vi "OnOff — копия.vi"(0 "setpoint":dbl step=0.01 format="%.2f", 1 "X1(SetState)":i32, 2 "reinitialize? (F)":bool, 5 "process variable":dbl step=0.01 format="%.2f", 7 "PID gains":T2={"proportional gain (Kc)"=1.0, "integral time (Ti, s)"=10.0, "derivative time (Td, s)"=1.0} {"derivative time (Td, s)" format="%.3f"; "integral time (Ti, s)" format="%.3f"; "proportional gain (Kc)" format="%.3f"}, 9 "manual control":dbl format="%.2f", 12 "output param":T1={"output high"=100.0, "alr value"=0.0, "output low"=0.0, "output rate (EGU/s)"=1.0, "dt (s)"=-1.0} {"dt (s)" format="%.3f"; "output rate (EGU/s)" format="%.2f"; "alr value" format="%.2f"; "output low" format="%.2f"; "output high" format="%.2f"}) -> (4 "output":dbl format="%.2f", 10 "dt out (s)":dbl format="%.3f")   [LabVIEW 2015]
uses:
  Userlib.lvlib
panel:
  # "Входы\nX1(SetState) заданное состояние\n     0 – аварийное значение\n     1 – минимум\n     2 – стоп\n     3 – ручной\n     4 – автомат\n     5 – максимум"
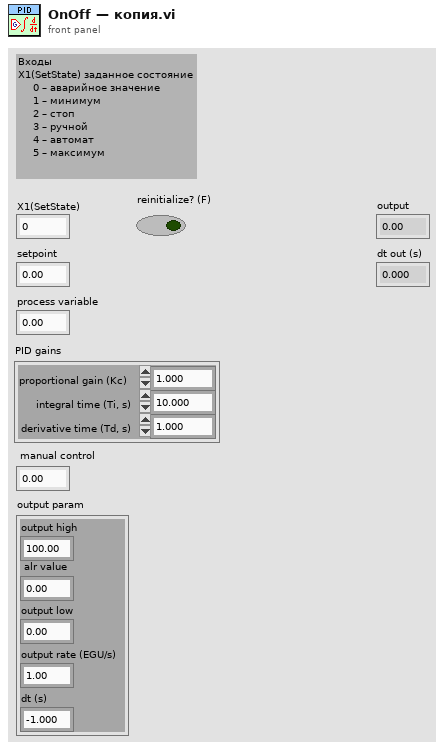
[diagram p1: front panel]
types:
  T1 = cluster{"output high":dbl, "alr value":dbl, "output low":dbl, "output rate (EGU/s)":dbl, "dt (s)":dbl}
  T2 = cluster{"proportional gain (Kc)":dbl, "integral time (Ti, s)":dbl, "derivative time (Td, s)":dbl}
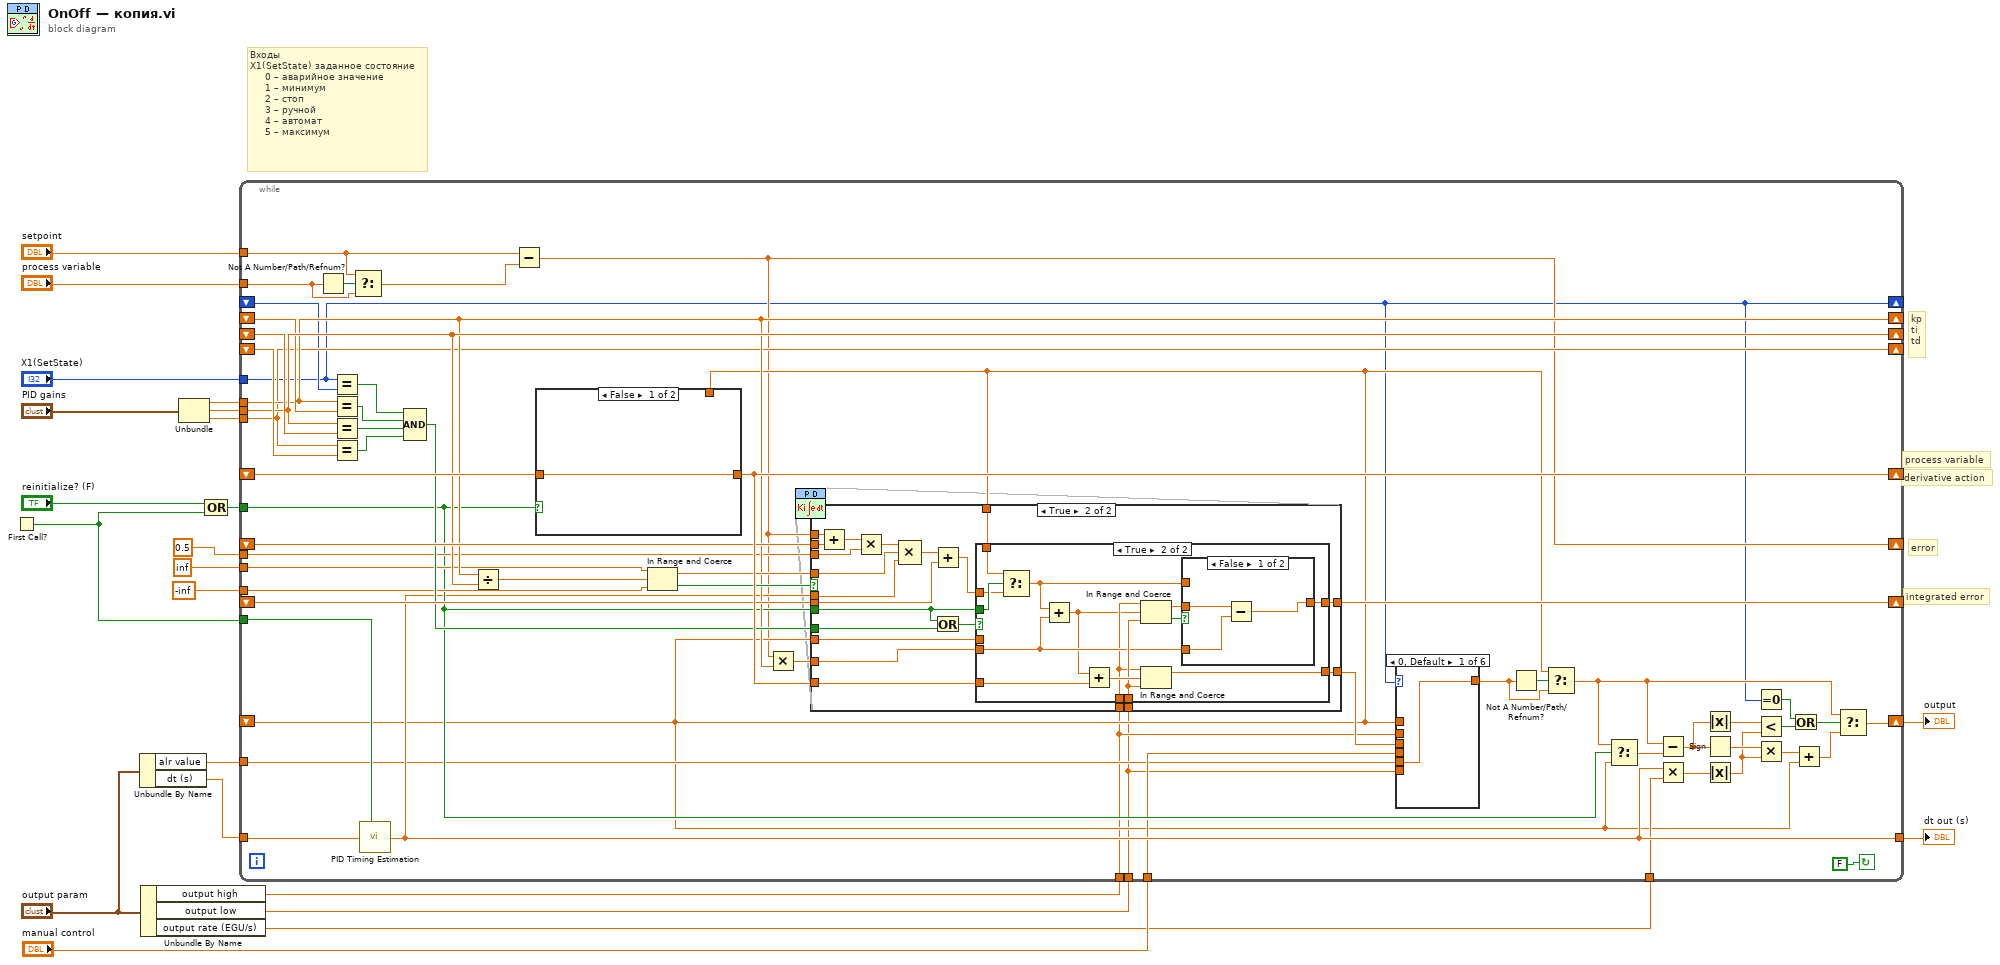
[diagram p0: block diagram]
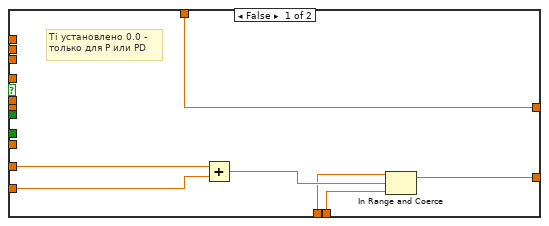
[diagram p2: hidden frame]
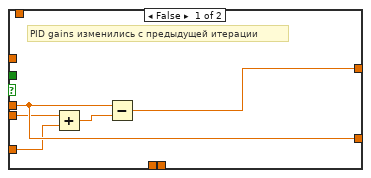
[diagram p3: hidden frame]
diagram:
  # "derivative action"
  # "process variable"
  # "kp\nti\ntd"
  # "error"
  # "integrated error"
  # "Входы\nX1(SetState) заданное состояние\n     0 – аварийное значение\n     1 – минимум\n     2 – стоп\n     3 – ручной\n     4 – автомат\n     5 – максимум"
  n1 = First Call?() -> (First Call?: T/F=w22:bool)
  n2 = Unbundle By Name("output param") -> ("alr value"=w6:dbl, "dt (s)"=w5:dbl)
  n3 = Unbundle By Name("output param") -> ("output high"=w14:dbl, "output low"=w15:dbl, "output rate (EGU/s)"=w1:dbl)
  n4 = Unbundle("PID gains") -> ("proportional gain (Kc)"=w11:dbl, "integral time (Ti, s)"=w12:dbl, "derivative time (Td, s)"=w13:dbl)
  n5 = Compound Arithmetic op=OR("reinitialize? (F)", w22) -> (w10:bool)
  n6 = while {
    tunnel: w10 -> [w49]
    shift-right: [w62] -> _
    shift-left: _ -> [w63]
    shift-right: [w64] -> _
    shift-left: _ -> [w78]
    shift-right: [w57] -> _
    shift-left: _ -> [w79]
    tunnel: w11 -> [w62]
    tunnel: w12 -> [w64]
    tunnel: w13 -> [w57]
    tunnel: w5 -> [w55]
    tunnel: w14 -> [w28]
    tunnel: w15 -> [w27]
    tunnel: "process variable" -> [w23]
    shift-right: [w74] -> _
    shift-left: _ -> [w68]
    shift-right: [w31] -> _
    shift-left: _ -> [w73]
    shift-right: [w72] -> _
    shift-left: _ -> [w71]
    tunnel: 0.5 ("y") -> [w61]
    tunnel: inf ("upper limit") -> [w59]
    tunnel: -inf ("lower limit") -> [w60]
    tunnel: w22 -> [w56]
    tunnel: [w48] -> w9
    tunnel: "manual control" -> [w38]
    tunnel: w1 -> [w47]
    shift-right: [w41] -> w7
    shift-left: _ -> [w34]
    tunnel: w6 -> [w36]
    tunnel: "X1(SetState)" -> [w29]
    shift-right: [w29] -> _
    shift-left: _ -> [w35]
    tunnel: "setpoint" -> [w24]
    stop <- FALSE continue-if-true
    n7 = Not A Number/Path/Refnum?(number/path/refnum=w23) -> (NaN/Path/Refnum?=w25:bool)
    n8 = Equal?(x=w29, y=w35) -> (x = y?=w30:bool)
    n9 = Equal?(x=w62, y=w63) -> (x = y?=w76:bool)
    n10 = Equal?(x=w64, y=w78) -> (x = y?=w75:bool)
    n11 = Equal?(x=w57, y=w79) -> (x = y?=w77:bool)
    n12 = Select(t=w24, s=w25, f=w23) -> (s? t:f=w26:dbl)
    n13 = call "PID Timing Estimation.vi"("R"=w56, "dt (s) in"=w55) -> ("dt (s) out"=w48:dbl)  [unwired: 7 in]
    n14 = Compound Arithmetic op=AND(w30, w76, w75, w77) -> (w65:bool)
    n15 = Divide(x=w62, y=w64) -> (x/y=w67:dbl)
    n16 = Subtract(x=w24, y=w26) -> (x-y=w31:dbl)
    n17 = case shown="False" w49 {
      tunnel: [w131 w132] -> w74
      tunnel: w68 -> [w131 _]
      tunnel: w34 -> [_ w132]
      frame False {
      }
      frame True {
      }
    }
    n18 = In Range and Coerce(upper limit=w59, x=w67, lower limit=w60) -> (coerced(x)=w70:dbl, In Range?=w69:bool)
    n19 = Multiply(x=w31, y=w62) -> (x*y=w66:dbl)
    n20 = case shown="True" w69 {
      tunnel: w31 -> [_ w106]
      tunnel: w73 -> [_ w107]
      tunnel: w71 -> [_ w102]
      tunnel: [w80 w97] -> w72
      tunnel: w70 -> [_ w95]
      tunnel: w66 -> [w85 w100]
      tunnel: [w86 w96] -> w39
      tunnel: w34 -> [_ w98]
      tunnel: w74 -> [w84 w94]
      tunnel: w49 -> [_ w93]
      tunnel: w65 -> [_ w92]
      tunnel: w48 -> [_ w91]
      tunnel: w28 -> [w82 w89]
      tunnel: w27 -> [w81 w90]
      tunnel: w61 -> [_ w88]
      tunnel: w34 -> [w80 w87]
      frame False {
        # "Ti установлено 0.0 -\nтолько для P или PD"
        n21 = Add(x=w85, y=w84) -> (x+y=w83:dbl)
        n22 = In Range and Coerce(upper limit=w82, x=w83, lower limit=w81) -> (coerced(x)=w86:dbl)  [unwired: 1 out]
      }
      frame True {
        n23 = Add(x=w106, y=w107) -> (x+y=w105:dbl)
        n24 = Multiply(x=w105, y=w88) -> (x*y=w104:dbl)
        n25 = Compound Arithmetic op=MULTIPLY(w104, w95, w91) -> (w103:dbl)
        n26 = Add(x=w103, y=w102) -> (x+y=w101:dbl)
        n27 = Or(x=w93, y=w92) -> (x .or. y?=w99:bool)
        n28 = case shown="True" w99 {
          tunnel: w101 -> [_ w113]
          tunnel: w100 -> [w110 w119]
          tunnel: w98 -> [w112 _]
          tunnel: w93 -> [_ w116]
          tunnel: [w111 w121] -> w97
          tunnel: [w112 w125] -> w96
          tunnel: w94 -> [w109 w124]
          tunnel: w90 -> [_ w123]
          tunnel: w89 -> [_ w118]
          tunnel: w87 -> [_ w115]
          frame False {
            # "PID gains изменились с предыдущей итерации"
            n29 = Add(x=w110, y=w109) -> (x+y=w108:dbl)
            n30 = Subtract(x=w112, y=w108) -> (x-y=w111:dbl)
          }
          frame True {
            n31 = Select(t=w115, s=w116, f=w113) -> (s? t:f=w114:dbl)
            n32 = Add(x=w114, y=w119) -> (x+y=w117:dbl)
            n33 = Add(x=w117, y=w124) -> (x+y=w126:dbl)
            n34 = In Range and Coerce(upper limit=w118, x=w117, lower limit=w123) -> (coerced(x)=w120:dbl, In Range?=w122:bool)
            n35 = In Range and Coerce(upper limit=w118, x=w126, lower limit=w123) -> (coerced(x)=w125:dbl)  [unwired: 1 out]
            n36 = case shown="False" w122 {
              tunnel: w114 -> [_ w130]
              tunnel: [w127 w130] -> w121
              tunnel: w120 -> [w129 _]
              tunnel: w119 -> [w128 _]
              frame False {
                n37 = Subtract(x=w129, y=w128) -> (x-y=w127:dbl)
              }
              frame True {
              }
            }
          }
        }
      }
    }
    n38 = case shown="0, Default" w29 {
      tunnel: w34 -> [_ _ w135 _ _ _]
      tunnel: w39 -> [_ _ _ _ w137 _]
      tunnel: w38 -> [_ _ _ w136 _ _]
      tunnel: [w133 w134 w135 w136 w137 w138] -> w37
      tunnel: w36 -> [w133 _ _ _ _ _]
      tunnel: w28 -> [_ _ _ _ _ w138]
      tunnel: w27 -> [_ w134 _ _ _ _]
      frame 0, Default {
      }
      frame 1 {
      }
      frame 2 {
      }
      frame 3 {
      }
      frame 4 {
      }
      frame 5 {
      }
    }
    n39 = Not A Number/Path/Refnum?(number/path/refnum=w37) -> (NaN/Path/Refnum?=w54:bool)
    n40 = Select(t=w34, s=w54, f=w37) -> (s? t:f=w40:dbl)
    n41 = Select(t=w40, s=w49, f=w34) -> (s? t:f=w45:dbl)
    n42 = Subtract(x=w40, y=w45) -> (x-y=w51:dbl)
    n43 = Multiply(x=w48, y=w47) -> (x*y=w53:dbl)
    n44 = Absolute Value(x=w51) -> (abs(x)=w43:dbl)
    n45 = Sign(1:w51) -> (0:w46:dbl)
    n46 = Absolute Value(x=w53) -> (abs(x)=w42:dbl)
    n47 = Equal To 0?(x=w29) -> (x = 0?=w32:bool)
    n48 = Less?(x=w43, y=w42) -> (x < y?=w52:bool)
    n49 = Multiply(x=w46, y=w42) -> (x*y=w44:dbl)
    n50 = Or(x=w32, y=w52) -> (x .or. y?=w33:bool)
    n51 = Add(x=w44, y=w34) -> (x+y=w50:dbl)
    n52 = Select(t=w40, s=w33, f=w50) -> (s? t:f=w41:dbl)
  }
  "output" <- w7
  "dt out (s)" <- w9
